vi "HFRR ADV v011 new software.vi"() -> ()   [LabVIEW 2025] (continued)
                    n2588 = call "file check.vi"("file name in"=w3137) -> ("error out"=w3140:errorcluster, "file name out"=w3135:string)  [unwired: 9 in]
                    n2589 = call "FILE PATH CREATION.vi"("error in"=w3140, "FILE NAME :"=w3135) -> ("FILE OUT"=w3138:path)  [unwired: 8 in, 1 out]
                    n2590 = Concatenate Strings(w3135, ".dgf" ("Substring")) -> (w3139:string)
                    n2591 = local read "FF 2"() -> (→"Frictional Force ( N )" →"Frictional Force ( N )":dbl)
                    n2592 = Build Path(base path=w3138, name or relative path=w3139) -> (appended path=w3134:path)
                    n2593 = local read "COF 2"() -> (w3148:dbl)
                    "cof" <- w3148
                    "Coefficient of Friction" <- w3148
                    "COF 4" <- w3148
                    "Coefficient of Friction" <- w3148
                    n2594 = local read "LVDT STROKE"() -> (w3132:dbl)
                    n2595 = local read "Add up Stroke"() -> (w3130:dbl)
                    n2596 = local read "TEMP"() -> (w3151:dbl)
                    "Temp" <- w3151
                    "Temperature ( Deg C )" <- w3151
                    n2597 = local read "Humidity ( %RH )"() -> (w3150:dbl)
                    "Humidity ( %RH )" <- w3150
                    "Humidity ( %RH )" <- w3150
                    n2598 = local read "Frequency ( Hz )"() -> (w3157:dbl)
                    n2599 = local read "Elapsed time"() -> (w3182:dbl)
                    n2600 = local read "AIR TEMP"() -> (w3155:dbl)
                    n2601 = local read "PID-out"() -> (w3160:dbl)
                    n2602 = Subtract(x=w3132, y=w3130) -> (x-y=w3131:dbl)
                    n2603 = Absolute Value(x=w3131) -> (abs(x)=w3129:dbl)
                    n2604 = local write "Temperature ( Deg C )"(w3151) -> ()
                    n2605 = Number To Fractional String(number=w3129, width (-)=i16 9 ("precision (6)"), precision (6)=i16 6) -> (F-format string=w3175:string)  [unwired: 1 in]
                    n2606 = Number To Fractional String(number=w3155, width (-)=i16 9 ("precision (6)"), precision (6)=i16 3) -> (F-format string=w3174:string)  [unwired: 1 in]
                    n2607 = Number To Fractional String(number=w3151, width (-)=i16 9 ("precision (6)"), precision (6)=i16 3) -> (F-format string=w3171:string)  [unwired: 1 in]
                    n2608 = Number To Fractional String(number=w3150, width (-)=i16 9 ("precision (6)"), precision (6)=i16 3) -> (F-format string=w3168:string)  [unwired: 1 in]
                    n2609 = Number To Fractional String(number=0.0, width (-)=i16 9 ("precision (6)"), precision (6)=i16 3) -> (F-format string=w3165:string)  [unwired: 1 in]
                    n2610 = Number To Fractional String(number=w3160, width (-)=i16 9 ("precision (6)"), precision (6)=i16 3) -> (F-format string=w3161:string)  [unwired: 1 in]
                    n2611 = Number To Fractional String(number=w3157, width (-)=i16 9 ("precision (6)"), precision (6)=i16 3) -> (F-format string=w3156:string)  [unwired: 1 in]
                    n2612 = Number To Fractional String(number=w3148, width (-)=i16 9 ("precision (6)"), precision (6)=i16 6) -> (F-format string=w3183:string)  [unwired: 1 in]
                    n2613 = Number To Fractional String(number=w3182, width (-)=i16 14 ("precision (6)"), precision (6)=i16 3) -> (F-format string=w3184:string)  [unwired: 1 in]
                    n2614 = Bundle("y"=1.02, w3129, "y"=0.98) -> (w3149:cluster{"y":dbl, dbl, "y":dbl})  [unwired: 1 in]
                    n2615 = Number To Fractional String(number="Ambient Humidity :", width (-)=i16 9 ("precision (6)"), precision (6)=i16 6) -> (F-format string=w3141:string)  [unwired: 1 in]
                    n2616 = local read "RUN"() -> (w3147:bool)
                    n2617 = case shown="True" w3147 {
                      tunnel: w3149 -> [_ w3194]
                      tunnel: w3129 -> [_ w3193]
                      tunnel: w3129 -> [_ w3191]
                      tunnel: w3129 -> [_ w3192]
                      frame False {
                      }
                      frame True {
                        "Stroke ( mm )" <- w3194
                        "Stroke ( mm )" <- w3194
                        "Stroke 4" <- w3193
                        "Stroke 3" <- w3191
                        "Stroke 2" <- w3192
                        "measured_stroke" <- w3191
                      }
                    }
                    n2618 = Concatenate Strings(w3184, w3143, w3183, w3143, w3175, w3143, w3174, w3143, w3171, w3143, w3168, w3143, w3165, w3143, w3161, w3143, w3156, w3143, w3141, "\r") -> (w3181:string)
                    n2619 = call <vilib>:"Write Characters To File.vi"("append to file? (new file:F)"=TRUE, "character string"=w3181, "file path (dialog if empty)"=w3134) -> ()  [unwired: 2 in, 1 out]
                    "refresh flag" <- TRUE ("refresh flag")
                  }
                }
                n2620 = case shown="True" w3054 {
                  tunnel: w3064 -> [_ w3090]
                  tunnel: w3069 -> [_ w3100]
                  tunnel: [0.0 w3096] -> _
                  tunnel: w3063 -> [_ w3095]
                  tunnel: [0.0 w3094] -> _
                  tunnel: w3053 -> [_ w3094]
                  tunnel: w3067 -> [w3083 _]
                  frame False {
                    n2621 = local write "acq timer"(w3083) -> ()
                    n2622 = local write "Test Duration Status"(0.0 ("Test Duration Status")) -> ()
                  }
                  frame True {
                    n2623 = local read "Set Hz"() -> (w3097:dbl)
                    n2624 = local write "Elapsed time"(w3090) -> ()
                    n2625 = local read "test time"() -> (w3089:dbl)
                    n2626 = Multiply(x=w3100, y=w3097) -> (x*y=w3099:dbl)
                    n2627 = case shown="False" w3095 {
                      tunnel: w3099 -> [w3101 _]
                      tunnel: [w3101 1.0] -> w3096
                      frame False {
                        n2628 = local write "Cycles elapsed"(w3101) -> ()
                      }
                      frame True {
                      }
                    }
                    n2629 = Greater?(x=w3090, y=w3089) -> (0:w3098:bool)
                    n2630 = Subtract(x=w3089, y=w3090) -> (x-y=w3088:dbl)
                    "time" <- w3088
                    n2631 = Multiply(x=w3088, y=60.0) -> (x*y=w3087:dbl)
                    n2632 = local write "Time Remaining"(w3087) -> ()
                    n2633 = local write "Remaining Time"(w3087) -> ()
                    n2634 = case shown="True" w3098 {
                      frame False {
                      }
                      frame True {
                        n2635 = stacked-sequence {
                          frame #0 {
                            w3106 = T17."Enabled" ("Disabled")
                            w3105 = FALSE ("TEST FILE NAM,E SAVED")
                            w3107 = "" ("FILE")
                            w3108 = TRUE ("Visible")
                            n2636 = local write "Humidity"(FALSE ("Humidity")) -> ()
                            n2637 = local write "RUN"(FALSE ("OK Button 2")) -> ()
                            n2638 = local write "Heater Button"(FALSE ("Heater Button")) -> ()
                            n2639 = local write "Auto Start Test"(FALSE ("Auto Start Test")) -> ()
                            n2640 = local write "TestCompFlg"(TRUE ("StpFlg")) -> ()
                            n2641 = local read "Humidity ( %RH )"() -> (→"Rh After":dbl)
                            n2642 = property on="STOP 2" class="Bool (strict)"("Disabled"=u8 0) -> ()  [unwired: 2 in, 2 out]
                            n2643 = local read "EVENT LOG"() -> (w3113:string)
                            n2644 = call "Event Log.vi"("Content"="Test Completed", "EVENT LOG"=w3113) -> ("EVENT LOG"=w3112:string)  [unwired: 8 in, 1 out]
                            n2645 = property on="RUN" class="Bool (strict)"("Visible"=w3108) -> ()  [unwired: 2 in, 2 out]
                            n2646 = property on="Auto Start Test" class="Bool (strict)"("Visible"=w3108) -> ()  [unwired: 2 in, 2 out]
                            n2647 = local write "Batch Ref Num :"(w3107) -> ()
                            n2648 = local write "FILE"(w3107) -> ()
                            n2649 = local write "EVENT LOG"(w3112) -> ()
                            n2650 = local write "TEST FILE NAM,E SAVED"(w3105) -> ()
                            n2651 = local write "Fuel Discription :"(w3107) -> ()
                            n2652 = local write "START TEMP"(w3105) -> ()
                            n2653 = local write "Remarks :"(w3107) -> ()
                            n2654 = local write "Main Dashboard Buttons"(T1."Imaging" ("Main Dashboard Buttons")) -> ()
                            n2655 = local write "Main Tab"(T2."Adv Scar" ("Main Tab")) -> ()
                            n2656 = property on="FRICVALZ 2" class="Bool (strict)"("DisabledEnum"=w3106) -> ()  [unwired: 2 in, 2 out]
                            n2657 = property on="FRICVALZ 3" class="Bool (strict)"("DisabledEnum"=w3106) -> ()  [unwired: 2 in, 2 out]
                            n2658 = property on="FRICVALZ 4" class="Bool (strict)"("DisabledEnum"=w3106) -> ()  [unwired: 2 in, 2 out]
                          }
                          frame #1 {
                            n2659 = Wait (ms)(milliseconds to wait=u32 1500) -> ()  [unwired: 1 out]
                          }
                          frame #2 {
                            n2660 = local write "Command"("VC;0") -> ()
                          }
                          frame #3 {
                            n2661 = Wait (ms)(milliseconds to wait=u32 1500) -> ()  [unwired: 1 out]
                          }
                          frame #4 {
                            n2662 = local write "Command"("VC;0") -> ()
                          }
                          frame #5 {
                            n2663 = Wait (ms)(milliseconds to wait=u32 1500) -> ()  [unwired: 1 out]
                          }
                          frame #6 {
                            n2664 = local write "Command"("ST;0") -> ()
                          }
                          frame #7 {
                            n2665 = local write "measured_stroke"(0.0 ("measured_stroke")) -> ()
                            n2666 = Wait (ms)(milliseconds to wait=u32 1500) -> ()  [unwired: 1 out]
                          }
                          frame #8 {
                            n2667 = local write "Command"("HE;0") -> ()
                          }
                        }
                      }
                    }
                    n2668 = Divide(x=w3090, y=w3089) -> (x/y=w3093:dbl)
                    n2669 = Multiply(x=w3093, y=100.0) -> (x*y=w3091:dbl)
                    n2670 = local write "Test Duration Status"(w3091) -> ()
                  }
                }
              }
              frame #2 {
                n2671 = case shown="True" "Heater Button" {
                  tunnel: [0.0 ("output") w3217] -> w3195
                  frame False {
                    w3198 = TRUE ("tmpchk")
                    n2672 = local read "TEMP"() -> (w3199:dbl)
                    n2673 = local write "Temp ini"(w3199) -> ()
                    n2674 = local write "Reset 4"(w3198) -> ()
                    n2675 = local write "tmpchk"(w3198) -> ()
                    n2676 = local write "reinit"(TRUE ("reinit")) -> ()
                    n2677 = local write "manual temp log"(TRUE ("manual temp log")) -> ()
                  }
                  frame True {
                    # "Logic to turn off\nthe heater when \ntemp is not rising.\nTime - 60 sec\nDelta t- 5°c"
                    n2678 = local read "Temp ini"() -> (w3206:dbl)
                    n2679 = local read "Auto Start Test"() -> (w3202:bool)
                    n2680 = Less?(x=w3206, y=53.0) -> (x < y?=w3204:bool)
                    n2681 = case shown="False" w3202 {
                      frame False {
                        n2682 = local read "Set Temp"() -> (w3226:dbl)
                        n2683 = local read "TEMP"() -> (w3225:dbl)
                        n2684 = Subtract(x=w3226, y=w3225) -> (x-y=w3224:dbl)
                        n2685 = Absolute Value(x=w3224) -> (abs(x)=w3223:dbl)
                        n2686 = Less?(x=w3223, y=0.5) -> (x < y?=w3221:bool)
                        n2687 = case shown="True" w3221 {
                          tunnel: "manual temp log" -> [_ w3227]
                          frame False {
                          }
                          frame True {
                            n2688 = case shown="True" w3227 {
                              selector: w3227 -> [_ w3228]
                              frame False {
                              }
                              frame True {
                                # "#Event log"
                                n2689 = Not(x=w3228) -> (.not. x?=w3229:bool)
                                n2690 = local write "manual temp log"(w3229) -> ()
                                n2691 = local read "EVENT LOG"() -> (w3232:string)
                                n2692 = call "Event Log.vi"("Content"="Target Temperature reached", "EVENT LOG"=w3232) -> ("EVENT LOG"=w3231:string)  [unwired: 8 in, 1 out]
                                n2693 = local write "EVENT LOG"(w3231) -> ()
                              }
                            }
                          }
                        }
                      }
                      frame True {
                        n2694 = local write "manual temp log"(TRUE ("manual temp log")) -> ()
                      }
                    }
                    n2695 = And(x="tmpchk", y=w3204) -> (x .and. y?=w3207:bool)
                    n2696 = case shown="True" w3207 {
                      frame False {
                      }
                      frame True {
                        n2697 = call "Elapsed Time8"("Time Target (s)"=300.0, "Reset"="Reset 4") -> ("Time has Elapsed"=w3234:bool)  [unwired: 10 in, 7 out]
                        n2698 = flat-sequence {
                          tunnel: w3234 -> [_]
                          frame #0 {
                            n2699 = local write "Reset 4"(FALSE ("Reset 4")) -> ()
                          }
                        }
                        n2700 = case shown="True" w3234 {
                          frame False {
                          }
                          frame True {
                            n2701 = local read "Temp ini"() -> (w3241:dbl)
                            n2702 = Add(x=w3241, y=5.0) -> (x+y=w3239:dbl)
                            n2703 = local read "TEMP"() -> (w3242:dbl)
                            n2704 = Greater?(x=w3242, y=w3239) -> (0:w3240:bool)
                            n2705 = case shown="False" w3240 {
                              frame False {
                                n2706 = local write "Heater Button"(FALSE ("Heater Button")) -> ()
                              }
                              frame True {
                                n2707 = local write "tmpchk"(FALSE ("tmpchk")) -> ()
                              }
                            }
                          }
                        }
                      }
                    }
                    n2708 = local read "Set Temp"() -> (w3215:dbl)
                    n2709 = local read "TEMP"() -> (w3209:dbl)
                    n2710 = call-poly <vilib>:"PID.vi"("reinitialize? (F)"="reinit", "dt (s)"=-1.0, "process variable"=w3209, "setpoint"=w3215) -> ("output"=w3212:dbl)  [unwired: 6 in, 1 out]
                    n2711 = Subtract(x=w3215, y=w3209) -> (x-y=w3216:dbl)
                    n2712 = Add(x=w3215, y=0.5) -> (x+y=w3213:dbl)
                    n2713 = Greater Or Equal?(x=w3209, y=w3213) -> ()  [unwired: 1 out]
                    n2714 = Select(t=0.0, s=FALSE, f=w3212) -> (s? t:f=w3211:dbl)
                    "PID output" <- w3211
                    n2715 = flat-sequence {
                      tunnel: w3211 -> [w3245]
                      tunnel: [w3245] -> w3217
                      frame #0 {
                        n2716 = local write "reinit"(FALSE ("reinit")) -> ()
                      }
                    }
                    n2717 = Bundle(w3216, "output"=w3211, "TEMP"=w3209) -> ()  [unwired: 1 in, 1 out]
                  }
                }
                "PID-out" <- w3195
              }
              frame #3 {
                n2718 = local read "TEMP"() -> (w3247:dbl)
                n2719 = Greater Or Equal?(x=w3247, y="Set Temp 2") -> (x >= y?=w3252:bool)
                n2720 = case shown="True" w3252 {
                  tunnel: [FALSE TRUE] -> w3250
                  frame False {
                  }
                  frame True {
                  }
                }
                "Status 13" <- w3250
                n2721 = And(x=w3250, y="trip1 8") -> (x .and. y?=w3249:bool)
                n2722 = case shown="True" w3249 {
                  frame False {
                    n2723 = local write "Heater Trip Temp"(TRUE ("Heater Trip Temp")) -> ()
                  }
                  frame True {
                    w3255 = FALSE ("OK Button 2")
                    n2724 = case shown="True" "Heater Trip Temp" {
                      selector: "Heater Trip Temp" -> [_ w3257]
                      frame False {
                      }
                      frame True {
                        n2725 = Not(x=w3257) -> (.not. x?=w3256:bool)
                        n2726 = local read "EVENT LOG"() -> (w3260:string)
                        n2727 = local write "Heater Trip Temp"(w3256) -> ()
                        n2728 = call "Event Log.vi"("Content"="Heater Trip", "EVENT LOG"=w3260) -> ("EVENT LOG"=w3259:string)  [unwired: 8 in, 1 out]
                        n2729 = local write "EVENT LOG"(w3259) -> ()
                      }
                    }
                    n2730 = local write "RUN"(w3255) -> ()
                    n2731 = property on="Auto Start Test" class="Bool (strict)"("Value"=w3255) -> ()  [unwired: 2 in, 2 out]
                    n2732 = local write "Heater Button"(w3255) -> ()
                  }
                }
              }
            }
            n2733 = case shown="False" w2978 {
              frame False {
                n2734 = disable-structure shown="Disabled" {
                  frame Disabled {
                    n2735 = stacked-sequence {
                      frame #0 {
                        n2736 = local write "RUN"(FALSE ("OK Button 2")) -> ()
                      }
                      frame #1 {
                      }
                    }
                  }
                  frame Enabled {
                  }
                }
              }
              frame True {
              }
            }
          }
        }
        n2737 = local read "airtempflg"() -> (w2770:bool)
        n2738 = Or(x=w2770, y=w2768) -> (x .or. y?=w2771:bool)
        n2739 = Insert Into Array(array=string[] ["Air Temperature has reached set value,", "Humidity has reached set value,", "Sample Temperaturehas reached set value,", ""], index=0, new element="") -> (w2756:string[])
        n2740 = Build Array(w2761, w2760, w2759) -> (w2757:i32[])
        n2741 = disable-structure shown="Disabled" {
          disable-tunnel: w2771 -> [w2848 _]
          disable-tunnel: w2766 -> [w2847 _]
          disable-tunnel: w2764 -> [w2846 _]
          frame Disabled {
            n2742 = Compound Arithmetic op=AND(w2848, w2847, w2846) -> ()  [unwired: 1 out]
            n2743 = case shown="True" {
              selector: _ -> [_ _]
              frame False {
              }
              frame True {
                w2849 = FALSE ("autostrtflg")
                n2744 = local write "RUN"(TRUE ("RUN")) -> ()
                n2745 = local write "autostrtflg"(w2849) -> ()
                n2746 = local write "autostart"(w2849) -> ()
                n2747 = local write "String 14"(" Running....." ("String 14")) -> ()
              }
            }
          }
          frame Enabled {
          }
        }
        n2748 = for {
          tunnel: w2757 -> [w2899] mode=indexing
          tunnel: w2756 -> [w2898]
          shift-right: [w2895] -> w2755
          shift-left: "" -> [w2897]
          n2749 = Index Array(array=w2898, index=w2899) -> (element=w2896:string)
          n2750 = Concatenate Strings(w2896, w2897) -> (w2895:string)
        }
        n2751 = local write "autostart 2"(w2755) -> ()
        n2752 = local read "Reset Graph"() -> (w2744:bool)
        n2753 = case shown="True" w2744 {
          selector: w2744 -> [_ w2798]
          frame False {
          }
          frame True {
            w2812 = 0.0 ("X Scale.Range:Maximum")
            n2754 = Not(x=w2798) -> (.not. x?=w2797:bool)
            n2755 = local write "Reset Graph"(w2797) -> ()
            n2756 = property on="Electrical Contact Resistance ( % )" class="WFChart (strict)"("XScale.Maximum"=600.0 ("X Scale.Range:Maximum"), "XScale.Minimum"=0.0 ("X Scale.Range:Minimum"), "YScale.Maximum"=100.0 ("Y Scale.Range:Maximum"), "YScale.Minimum"=0.0 ("Y Scale.Range:Minimum")) -> ()  [unwired: 2 in, 2 out]
            n2757 = property on="Frictional Force ( N )" class="WFChart (strict)"("XScale.Maximum"=600.0 ("X Scale.Range:Maximum"), "XScale.Minimum"=0.0 ("X Scale.Range:Minimum"), "YScale.Maximum"=100.0 ("Y Scale.Range:Maximum"), "YScale.Minimum"=0.0 ("Y Scale.Range:Minimum")) -> ()  [unwired: 2 in, 2 out]
            n2758 = property on="Temperature ( Deg C )" class="WFChart (strict)"("XScale.Maximum"=600.0 ("X Scale.Range:Maximum"), "XScale.Minimum"=0.0 ("X Scale.Range:Minimum"), "YScale.Maximum"=100.0 ("Y Scale.Range:Maximum"), "YScale.Minimum"=0.0 ("Y Scale.Range:Minimum")) -> ()  [unwired: 2 in, 2 out]
            n2759 = property on="Humidity ( %RH )" class="WFChart (strict)"("XScale.Maximum"=600.0 ("X Scale.Range:Maximum"), "XScale.Minimum"=0.0 ("X Scale.Range:Minimum"), "YScale.Maximum"=100.0 ("Y Scale.Range:Maximum"), "YScale.Minimum"=0.0 ("Y Scale.Range:Minimum")) -> ()  [unwired: 2 in, 2 out]
            n2760 = property on="Stroke ( mm )" class="WFChart (strict)"("XScale.Maximum"=600.0 ("X Scale.Range:Maximum"), "XScale.Minimum"=0.0 ("X Scale.Range:Minimum"), "YScale.Maximum"=100.0 ("Y Scale.Range:Maximum"), "YScale.Minimum"=0.0 ("Y Scale.Range:Minimum")) -> ()  [unwired: 2 in, 2 out]
            n2761 = property on="Coefficient of Friction" class="WFChart (strict)"("XScale.Maximum"=600.0 ("X Scale.Range:Maximum"), "XScale.Minimum"=0.0 ("X Scale.Range:Minimum"), "YScale.Maximum"=100.0 ("Y Scale.Range:Maximum"), "YScale.Minimum"=0.0 ("Y Scale.Range:Minimum")) -> ()  [unwired: 2 in, 2 out]
            n2762 = property on="Electrical Contact Resistance ( % )" class="WFChart (strict)"("XScale.Minimum"=0.0 ("X Scale.Range:Minimum"), "XScale.Maximum"=600.0 ("X Scale.Range:Maximum"), "YScale.Minimum"=0.0 ("Y Scale.Range:Minimum"), "YScale.Maximum"=100.0 ("Y Scale.Range:Maximum")) -> ()  [unwired: 2 in, 2 out]
            n2763 = property on="Temperature ( Deg C )" class="WFChart (strict)"("XScale.Minimum"=0.0 ("X Scale.Range:Minimum"), "XScale.Maximum"=600.0 ("X Scale.Range:Maximum"), "YScale.Minimum"=0.0 ("Y Scale.Range:Minimum"), "YScale.Maximum"=100.0 ("Y Scale.Range:Maximum")) -> ()  [unwired: 2 in, 2 out]
            n2764 = property on="Coefficient of Friction" class="WFChart (strict)"("XScale.Minimum"=0.0 ("X Scale.Range:Minimum"), "XScale.Maximum"=600.0 ("X Scale.Range:Maximum"), "YScale.Maximum"=1.0 ("X Scale.Range:Minimum"), "YScale.Minimum"=0.0 ("X Scale.Range:Minimum")) -> ()  [unwired: 2 in, 2 out]
            n2765 = property on="Frictional Force ( N )" class="WFChart (strict)"("XScale.Maximum"=600.0 ("X Scale.Range:Maximum"), "XScale.Minimum"=w2812, "YScale.Maximum"=10.0 ("Y Scale.Range:Maximum"), "YScale.Minimum"=w2812) -> ()  [unwired: 2 in, 2 out]
            n2766 = property on="Stroke ( mm )" class="WFChart (strict)"("XScale.Maximum"=600.0 ("X Scale.Range:Maximum"), "XScale.Minimum"=0.0 ("X Scale.Range:Minimum"), "YScale.Maximum"=100.0 ("Y Scale.Range:Maximum"), "YScale.Minimum"=0.0 ("Y Scale.Range:Minimum")) -> ()  [unwired: 2 in, 2 out]
            n2767 = property on="Humidity ( %RH )" class="WFChart (strict)"("XScale.Maximum"=600.0 ("X Scale.Range:Maximum"), "XScale.Minimum"=0.0 ("X Scale.Range:Minimum"), "YScale.Maximum"=100.0 ("Y Scale.Range:Maximum"), "YScale.Minimum"=0.0 ("Y Scale.Range:Minimum")) -> ()  [unwired: 2 in, 2 out]
          }
        }
      }
      frame "Compare Files" {
        # "Elapsed time\ncof\nstroke\nAir temp\nTemp\nHumidity"
        n2768 = case shown="True" "RSTV1 2" {
          frame False {
          }
          frame True {
            n2769 = property on="Humidity ( %RH )" class="XYGraph (strict)"("Y Scale.Display Format:Precision"=u8 0 ("Y Scale.Format & Precision:Precision")) -> ()  [unwired: 2 in, 2 out]
            n2770 = property on="Humidity ( %RH )" class="XYGraph (strict)"("X Scale.Range:Minimum"=0.0, "X Scale.Range:Maximum"=75.0, "Y Scale.Range:Minimum"=48.0, "Y Scale.Range:Maximum"=58.0) -> ()  [unwired: 2 in, 2 out]
          }
        }
        n2771 = case shown="True" "RST CP 2" {
          frame False {
          }
          frame True {
            n2772 = property on="XY Graph 13" class="XYGraph (strict)"("Y Scale.Display Format:Precision"=u8 0 ("Y Scale.Format & Precision:Precision")) -> ()  [unwired: 2 in, 2 out]
            n2773 = property on="XY Graph 13" class="XYGraph (strict)"("X Scale.Range:Minimum"=0.0, "X Scale.Range:Maximum"=75.0, "Y Scale.Range:Minimum"=0.0, "Y Scale.Range:Maximum"=100.0) -> ()  [unwired: 2 in, 2 out]
          }
        }
        n2774 = case shown="True" "RST CP" {
          frame False {
          }
          frame True {
            n2775 = property on="Sample Temperature ( °C )" class="XYGraph (strict)"("Y Scale.Display Format:Precision"=u8 2 ("Y Scale.Format & Precision:Precision")) -> ()  [unwired: 2 in, 2 out]
            n2776 = property on="Sample Temperature ( °C )" class="XYGraph (strict)"("X Scale.Range:Minimum"=0.0, "X Scale.Range:Maximum"=75.0, "Y Scale.Range:Minimum"=58.0, "Y Scale.Range:Maximum"=62.0) -> ()  [unwired: 2 in, 2 out]
          }
        }
        n2777 = case shown="True" "RSTV1 3" {
          frame False {
          }
          frame True {
            n2778 = property on="Air Temperature  ( °C )" class="XYGraph (strict)"("Y Scale.Display Format:Precision"=u8 2 ("Y Scale.Format & Precision:Precision")) -> ()  [unwired: 2 in, 2 out]
            n2779 = property on="Air Temperature  ( °C )" class="XYGraph (strict)"("X Scale.Range:Minimum"=0.0 ("Y Scale.Range:Minimum"), "X Scale.Range:Maximum"=75.0 ("Y Scale.Range:Maximum"), "Y Scale.Range:Minimum"=20.0 ("X Scale.Range:Minimum"), "Y Scale.Range:Maximum"=26.0 ("X Scale.Range:Maximum")) -> ()  [unwired: 2 in, 2 out]
          }
        }
        n2780 = case shown="True" "RSTV1 4" {
          frame False {
          }
          frame True {
            n2781 = property on="Stroke ( mm )" class="XYGraph (strict)"("Y Scale.Display Format:Precision"=u8 2 ("Y Scale.Format & Precision:Precision")) -> ()  [unwired: 2 in, 2 out]
            n2782 = property on="Stroke ( mm )" class="XYGraph (strict)"("X Scale.Range:Minimum"=0.0 ("Y Scale.Range:Maximum"), "X Scale.Range:Maximum"=75.0 ("X Scale.Range:Minimum"), "Y Scale.Range:Minimum"=0.98, "Y Scale.Range:Maximum"=1.02) -> ()  [unwired: 2 in, 2 out]
          }
        }
        n2783 = case shown="True" "rstv2" {
          frame False {
          }
          frame True {
            n2784 = property on="Coefficient Of Friction" class="XYGraph (strict)"("Y Scale.Display Format:Precision"=u8 3 ("Y Scale.Format & Precision:Precision")) -> ()  [unwired: 2 in, 2 out]
            n2785 = property on="Coefficient Of Friction" class="XYGraph (strict)"("X Scale.Range:Minimum"=0.0 ("Y Scale.Range:Maximum"), "X Scale.Range:Maximum"=75.0, "Y Scale.Range:Minimum"=0.0, "Y Scale.Range:Maximum"=1.0 ("X Scale.Range:Minimum")) -> ()  [unwired: 2 in, 2 out]
          }
        }
        n2786 = case shown="True" "RST CP 3" {
          frame False {
          }
          frame True {
            n2787 = property on="Air Temp ( °C ) vs Humidity ( % RH )" class="XYGraph (strict)"("X Scale.Range:Minimum"=18.0, "X Scale.Range:Maximum"=28.0 ("X Scale.Range:Minimum"), "Y Scale.Range:Minimum"=30.0 ("X Scale.Range:Minimum"), "Y Scale.Range:Maximum"=70.0 ("X Scale.Range:Minimum")) -> ()  [unwired: 2 in, 2 out]
          }
        }
        n2788 = case shown="True" "OPEN 1" {
          frame False {
          }
          frame True {
            (unwired) 0  # existing file
            w3536 = "Choose a datalog file to open"  # prompt
            n2789 = local write "OPEN 1"(FALSE ("OPEN 1")) -> ()
            n2790 = String To Path(string="C:\\LAB-IQ\\Data\\") -> (path=w3521:path)
            n2791 = File Dialog(6:"*.dgf" ("pattern"), 7:w3536, 11:w3521) -> (0:w3519:errorcluster, 3:w3527:path)  [unwired: 4 in, 2 out]
            n2792 = Unbundle(w3519) -> ()  [unwired: 3 out]
            n2793 = Strip Path(path=w3527) -> (name=w3526:string)  [unwired: 1 out]
            n2794 = Path To String(path=w3527) -> (string=w3522:string)
            "string1" <- w3522
            n2795 = Match Pattern(string=w3526, regular expression=".dgf") -> (before substring=→"String Control":string)  [unwired: 1 in, 3 out]
            n2796 = Match Pattern(string=w3522, regular expression=".dgf" ("substring (\"\")")) -> (before substring=w3532:string)  [unwired: 1 in, 3 out]
            n2797 = Concatenate Strings(w3532, ".duf" ("Substring")) -> (w3528:string)
            n2798 = String To Path(string=w3528) -> (path=w3533:path)
            n2799 = call <vilib>:"Read Characters From File.vi"("file path (dialog if empty)"=w3533, "start of read offset (chars.:0)"=60 ("start of read offset (chars.: 0)")) -> ("character string"=→"String Control 2":string)  [unwired: 4 in, 3 out]
          }
        }
        n2800 = case shown="True" "OPEN 2" {
          frame False {
          }
          frame True {
            (unwired) 0  # existing file
            w3554 = "Choose a datalog file to open"  # prompt
            n2801 = local write "OPEN 2"(FALSE ("OPEN 1")) -> ()
            n2802 = String To Path(string="C:\\LAB-IQ\\Data\\") -> (path=w3539:path)
            n2803 = File Dialog(6:"*.dgf" ("pattern"), 7:w3554, 11:w3539) -> (0:w3537:errorcluster, 3:w3545:path)  [unwired: 4 in, 2 out]
            n2804 = Unbundle(w3537) -> ()  [unwired: 3 out]
            n2805 = Strip Path(path=w3545) -> (name=w3543:string)  [unwired: 1 out]
            n2806 = Path To String(path=w3545) -> (string=w3540:string)
            "string1 2" <- w3540
            n2807 = Match Pattern(string=w3543, regular expression=".dgf") -> (before substring=→"String Control 3":string)  [unwired: 1 in, 3 out]
            n2808 = Match Pattern(string=w3540, regular expression=".dgf" ("substring (\"\")")) -> (before substring=w3551:string)  [unwired: 1 in, 3 out]
            n2809 = Concatenate Strings(w3551, ".duf" ("Substring")) -> (w3548:string)
            n2810 = String To Path(string=w3548) -> (path=w3546:path)
            n2811 = call <vilib>:"Read Characters From File.vi"("file path (dialog if empty)"=w3546, "start of read offset (chars.:0)"=60 ("start of read offset (chars.: 0)")) -> ("character string"=→"String Control 4":string)  [unwired: 4 in, 3 out]
          }
        }
        n2812 = case shown="True" "OPEN 3" {
          frame False {
          }
          frame True {
            (unwired) 0  # existing file
            w3572 = "Choose a datalog file to open"  # prompt
            n2813 = local write "OPEN 3"(FALSE ("OPEN 1")) -> ()
            n2814 = String To Path(string="C:\\LAB-IQ\\Data\\") -> (path=w3557:path)
            n2815 = File Dialog(6:"*.dgf" ("pattern"), 7:w3572, 11:w3557) -> (0:w3555:errorcluster, 3:w3563:path)  [unwired: 4 in, 2 out]
            n2816 = Unbundle(w3555) -> ()  [unwired: 3 out]
            n2817 = Strip Path(path=w3563) -> (name=w3561:string)  [unwired: 1 out]
            n2818 = Path To String(path=w3563) -> (string=w3558:string)
            "string1 3" <- w3558
            n2819 = Match Pattern(string=w3561, regular expression=".dgf") -> (before substring=→"String Control 5":string)  [unwired: 1 in, 3 out]
            n2820 = Match Pattern(string=w3558, regular expression=".dgf" ("substring (\"\")")) -> (before substring=w3568:string)  [unwired: 1 in, 3 out]
            n2821 = Concatenate Strings(w3568, ".duf" ("Substring")) -> (w3565:string)
            n2822 = String To Path(string=w3565) -> (path=w3569:path)
            n2823 = call <vilib>:"Read Characters From File.vi"("file path (dialog if empty)"=w3569, "start of read offset (chars.:0)"=60 ("start of read offset (chars.: 0)")) -> ("character string"=→"String Control 6":string)  [unwired: 4 in, 3 out]
          }
        }
        n2824 = case shown="True" "OPEN 4" {
          frame False {
          }
          frame True {
            (unwired) 0  # existing file
            w3590 = "Choose a datalog file to open"  # prompt
            n2825 = local write "OPEN 4"(FALSE ("OPEN 1")) -> ()
            n2826 = String To Path(string="C:\\LAB-IQ\\Data\\") -> (path=w3575:path)
            n2827 = File Dialog(6:"*.dgf" ("pattern"), 7:w3590, 11:w3575) -> (0:w3573:errorcluster, 3:w3581:path)  [unwired: 4 in, 2 out]
            n2828 = Unbundle(w3573) -> ()  [unwired: 3 out]
            n2829 = Strip Path(path=w3581) -> (name=w3579:string)  [unwired: 1 out]
            n2830 = Path To String(path=w3581) -> (string=w3576:string)
            "string1 4" <- w3576
            n2831 = Match Pattern(string=w3579, regular expression=".dgf") -> (before substring=→"String Control 7":string)  [unwired: 1 in, 3 out]
            n2832 = Match Pattern(string=w3576, regular expression=".dgf" ("substring (\"\")")) -> (before substring=w3586:string)  [unwired: 1 in, 3 out]
            n2833 = Concatenate Strings(w3586, ".duf" ("Substring")) -> (w3583:string)
            n2834 = String To Path(string=w3583) -> (path=w3587:path)
            n2835 = call <vilib>:"Read Characters From File.vi"("file path (dialog if empty)"=w3587, "start of read offset (chars.:0)"=60 ("start of read offset (chars.: 0)")) -> ("character string"=→"String Control 8":string)  [unwired: 4 in, 3 out]
          }
        }
      }
      frame "About" {
        # "Elapsed time\ncof\nstroke\nmean pos\nTemp\nHumidity"
        n2836 = disable-structure shown="Disabled" {
          frame Disabled {
            n2837 = case shown="True" "Export" {
              frame False {
              }
              frame True {
                w3612 = "                                      " ("string")
                w3614 = "\r"
                (unwired) i16 6 ("width (-)")
                w3691 = "\r"
                w3623 = "\r"
                n2838 = local write "Export"(FALSE ("Export")) -> ()
                n2839 = local read "String 29"() -> (w3660:string)
                n2840 = local read "String 34"() -> (w3648:string)
                n2841 = local read "String 35"() -> (w3643:string)
                n2842 = local read "String 37"() -> (w3639:string)
                n2843 = local read "String 36"() -> (w3636:string)
                n2844 = local read "String 38"() -> (w3633:string)
                n2845 = local read "String 39"() -> (w3630:string)
                n2846 = Match Pattern(string=w3660, regular expression=".dwm") -> (before substring=w3656:string)  [unwired: 1 in, 3 out]
                "before substring" <- w3656
                n2847 = local read "S 38"() -> (w3651:string)
                n2848 = local read "S 39"() -> (w3644:string)
                n2849 = local read "Temperature before test 2"() -> (w3680:dbl)
                n2850 = local read "Temperature after test 2"() -> (w3685:dbl)
                n2851 = local read "Humidity before test 2"() -> (w3666:dbl)
                n2852 = local read "Humidity after test 2"() -> (w3681:dbl)
                n2853 = local read "MWSD 2"() -> (w3677:dbl)
                n2854 = local read "WS1.4 2"() -> (w3693:dbl)
                n2855 = local read "HCF 2"() -> (w3689:dbl)
                n2856 = local read "AVP 2"() -> (w3678:dbl)
                n2857 = Concatenate Strings("1," ("string"), w3651) -> (w3650:string)
                n2858 = Concatenate Strings("2," ("string"), w3648) -> (w3647:string)
                n2859 = Concatenate Strings("3," ("string"), w3644) -> (w3646:string)
                n2860 = Concatenate Strings("4," ("string"), w3643) -> (w3642:string)
                n2861 = Concatenate Strings("5," ("string"), w3639) -> (w3640:string)
                n2862 = Concatenate Strings("6," ("string"), w3636) -> (w3637:string)
                n2863 = Concatenate Strings("7," ("string"), w3633) -> (w3634:string)
                n2864 = Concatenate Strings("8," ("string"), w3630) -> (w3631:string)
                n2865 = local read "Sample ID"() -> (w3698:string)
                n2866 = case shown="\"xlx\"" "Select File Type" {
                  tunnel: w3656 -> [w3701 w3703 w3705]
                  tunnel: [w3699 w3704 w3706] -> w3655
                  frame "xlx" {
                    n2867 = Concatenate Strings(w3701, ".xls" ("string")) -> (w3699:string)
                  }
                  frame "csv" {
                    n2868 = Concatenate Strings(w3703, ".csv" ("string")) -> (w3704:string)
                  }
                  frame "txt" {
                    n2869 = Concatenate Strings(w3705, ".txt" ("string")) -> (w3706:string)
                  }
                }
                n2870 = local read "Test Date"() -> (w3697:string)
                n2871 = local read "String 45"() -> (w3611:string)
                n2872 = local read "String 31"() -> (w3696:string)
                n2873 = local read "String 32"() -> (w3695:string)
                n2874 = local read "TITTLE"() -> (w3619:string)
                n2875 = Number To Fractional String(number=w3666, width (-)=i16 6, precision (6)=i16 2) -> (F-format string=w3665:string)  [unwired: 1 in]
                n2876 = Number To Fractional String(number=w3680, width (-)=i16 6, precision (6)=i16 2) -> (F-format string=w3686:string)  [unwired: 1 in]
                n2877 = Number To Fractional String(number=w3681, width (-)=i16 6, precision (6)=i16 2) -> (F-format string=w3679:string)  [unwired: 1 in]
                n2878 = Number To Fractional String(number=w3685, width (-)=i16 6, precision (6)=i16 2) -> (F-format string=w3684:string)  [unwired: 1 in]
                n2879 = Number To Fractional String(number=w3677, width (-)=i16 6, precision (6)=i16 2) -> (F-format string=w3675:string)  [unwired: 1 in]
                n2880 = Number To Fractional String(number=w3678, width (-)=i16 6, precision (6)=i16 2) -> (F-format string=w3676:string)  [unwired: 1 in]
                n2881 = Number To Fractional String(number=w3689, width (-)=i16 6, precision (6)=i16 2) -> (F-format string=w3690:string)  [unwired: 1 in]
                n2882 = Number To Fractional String(number=w3693, precision (6)=i16 2) -> (F-format string=w3694:string)  [unwired: 2 in]
                n2883 = local read "s.NO"() -> (w3613:string)
                n2884 = Concatenate Strings("=" ("string"), w3619) -> (w3618:string)
                n2885 = Concatenate Strings("S.No," ("string"), "                                       Parameters" ("string")) -> (w3624:string)
                n2886 = Concatenate Strings(w3691, w3650, w3665, w3691, w3647, w3686, w3691, w3646, w3679, w3691, w3642, w3684, w3691, w3640, w3675, w3691, w3637, w3676, w3691, w3634, w3690, w3691, w3631, w3694) -> (w3653:string)
                n2887 = Concatenate Strings(w3623, "," ("string"), w3611, w3613, w3612, w3695, w3698, w3612, w3696, w3697, w3623) -> (w3621:string)
                n2888 = local read "Tested by"() -> (w3627:string)
                n2889 = local read "String 33"() -> (w3628:string)
                n2890 = Concatenate Strings("," ("string"), "                                                                             " ("string")) -> (w3616:string)
                n2891 = Concatenate Strings(w3618, w3614, w3621, w3614, w3624, w3653, w3614, w3616, w3628, w3627) -> (→"export":string)
                n2892 = String To Path(string=w3655) -> (path=w3662:path)
                n2893 = local read "export"() -> (w3657:string)
                n2894 = call <vilib>:"Write Characters To File.vi"("append to file? (new file:F)"=FALSE, "character string"=w3657, "file path (dialog if empty)"=w3662) -> ()  [unwired: 2 in, 1 out]
              }
            }
          }
          frame Enabled {
          }
        }
        n2895 = case shown="True" "OK Button 17" {
          frame False {
          }
          frame True {
            (unwired) 0  # existing file
            w3915 = "Choose a datalog file to open"  # prompt
            n2896 = local write "OK Button 17"(FALSE ("OK Button 17")) -> ()
            n2897 = local read "String"() -> (w3910:string)
            n2898 = String To Path(string=w3910) -> (path=w3911:path)
            n2899 = File Dialog(6:"*.duf" ("pattern"), 7:w3915, 11:w3911) -> (0:w3902:errorcluster, 3:w3921:path)  [unwired: 4 in, 2 out]
            n2900 = Unbundle(w3902) -> ()  [unwired: 3 out]
            n2901 = Open/Create/Replace File "Open File"(file path (use dialog)=w3921) -> (refnum out=w3913:refnum<file>)  [unwired: 5 in, 2 out]
            n2902 = Strip Path(path=w3921) -> (name=w3919:string)  [unwired: 1 out]
            n2903 = Path To String(path=w3921) -> (string=w3904:string)
            n2904 = while {
              tunnel: w3913 -> [w3925]
              i -> [w3922]
              stop <- w3923 continue-if-true
              (unwired) TRUE ("line mode (F)")
              n2905 = Read from Text File "Read File"(file (use dialog)=w3925) -> (text=w3924:string)  [unwired: 3 in, 3 out]
              n2906 = local write "Numeric 16"(w3922) -> ()
              n2907 = String Length(string=w3924) -> (length=w3927:i32)
              n2908 = Greater?(x=w3927, y=1) -> (0:w3923:bool)
            }
            n2909 = local write "String 29"(w3904) -> ()
            n2910 = Search and Replace String(input string=w3904, search string=".duf", replace string=".dgf" ("replace string (\"\")")) -> (result string=→"String Indicator 4":string)  [unwired: 5 in, 3 out]
            n2911 = Match Pattern(string=w3919, regular expression=".dwm") -> (before substring=w3903:string)  [unwired: 1 in, 3 out]
            "String Indicator" <- w3903
            n2912 = Match Pattern(string=w3904, regular expression=".dwm" ("substring (\"\")")) -> (before substring=w3905:string)  [unwired: 1 in, 3 out]
            "String Indicator 3" <- w3905
            n2913 = local write "TITTLE 2"(w3903) -> ()
            n2914 = String To Path(string=w3905) -> (path=w3912:path)
            "path" <- w3912
            n2915 = call <vilib>:"Read Characters From File.vi"("file path (dialog if empty)"=w3912, "start of read offset (chars.:0)"=60 ("start of read offset (chars.: 0)")) -> ("character string"=→"String Indicator 2":string)  [unwired: 4 in, 3 out]
          }
        }
        n2916 = call <vilib>:"Query Available Printers.vi"() -> ("system configured printers"=w3604:string[])  [unwired: 9 in, 2 out]
        "System Configured Printers 2" <- w3604
        n2917 = local read "OK Button 16"() -> (w3601:bool)
        n2918 = case shown="True" "OK Button 16" {
          frame False {
          }
          frame True {
            n2919 = stacked-sequence {
              frame #0 {
                n2920 = local read "Numeric 16"() -> (w3929:i32)
                n2921 = local write "Numeric 10"(w3929) -> ()
              }
              frame #1 {
                n2922 = local read "S.NO"() -> (→"s.NO":string)
                n2923 = local read "String 29"() -> (w3933:string)
                n2924 = String To Path(string=w3933) -> (path=w3932:path)
                n2925 = Open/Create/Replace File "Open File"(file path (use dialog)=w3932) -> (refnum out=w3934:refnum<file>)  [unwired: 5 in, 2 out]
                n2926 = for {
                  N: 16 -> [_]
                  tunnel: w3934 -> [w3941]
                  i -> [w3937]
                  (unwired) TRUE ("line mode (F)")
                  n2927 = Read from Text File "Read File"(file (use dialog)=w3941) -> (text=w3935:string)  [unwired: 3 in, 3 out]
                  n2928 = Match Pattern(string=w3935, regular expression="(") -> (after substring=w3940:string)  [unwired: 1 in, 3 out]
                  n2929 = Match Pattern(string=w3940, regular expression=")") -> (before substring=w3936:string)  [unwired: 1 in, 3 out]
                  n2930 = case shown="1" w3937 {
                    tunnel: w3936 -> [w3942 w3943 _ _ w3944 w3945 w3946 w3948 w3950 w3952 w3954 w3956 w3958 w3960 _]
                    tunnel: w3935 -> [_ _ _ _ _ _ _ _ _ _ _ _ _ _ _]
                    frame 0 {
                      "TITTLE" <- w3942
                    }
                    frame 1 {
                      "Sample ID" <- w3943
                    }
                    frame 2 {
                    }
                    frame 3 {
                    }
                    frame 4 {
                      "Test Date" <- w3944
                    }
                    frame 5 {
                      "Tested by" <- w3945
                    }
                    frame 6 {
                      n2931 = Fract/Exp String To Number(string=w3946) -> (number=→"Humidity before test 2":dbl)  [unwired: 3 in, 1 out]
                    }
                    frame 7 {
                      n2932 = Fract/Exp String To Number(string=w3948) -> (number=→"Temperature before test 2":dbl)  [unwired: 3 in, 1 out]
                    }
                    frame 8 {
                      n2933 = Fract/Exp String To Number(string=w3950) -> (number=→"Humidity after test 2":dbl)  [unwired: 3 in, 1 out]
                    }
                    frame 9 {
                      n2934 = Fract/Exp String To Number(string=w3952) -> (number=→"Temperature after test 2":dbl)  [unwired: 3 in, 1 out]
                    }
                    frame 10 {
                      n2935 = Fract/Exp String To Number(string=w3954) -> (number=→"MWSD 2":dbl)  [unwired: 3 in, 1 out]
                    }
                    frame 11 {
                      n2936 = Fract/Exp String To Number(string=w3956) -> (number=→"AVP 2":dbl)  [unwired: 3 in, 1 out]
                    }
                    frame 12 {
                      n2937 = Fract/Exp String To Number(string=w3958) -> (number=→"HCF 2":dbl)  [unwired: 3 in, 1 out]
                    }
                    frame 13 {
                      n2938 = Fract/Exp String To Number(string=w3960) -> (number=→"WS1.4 2":dbl)  [unwired: 3 in, 1 out]
                    }
                    frame 14, Default {
                    }
                  }
                }
              }
              frame #2 {
              }
            }
            n2939 = local write "OK Button 16"(FALSE ("OK Button 13")) -> ()
          }
        }
        n2940 = Index Array(array=w3604, index="Select Printer 3") -> (element=w3606:string)
        "Selected Printer" <- w3606
        n2941 = case shown="True" w3601 {
          frame False {
          }
          frame True {
            n2942 = flat-sequence {
              frame #0 {
              }
              frame #1 {
                n2943 = Wait (ms)(milliseconds to wait=u32 100) -> ()  [unwired: 1 out]
              }
              frame #2 {
                n2944 = local write "OK Button 16"(FALSE ("Print 3")) -> ()
              }
            }
          }
        }
        n2945 = case shown="True" "Print" {
          tunnel: w3606 -> [_ w3898]
          frame False {
          }
          frame True {
            (unwired) i16 6 ("width (-)")
            (unwired) "TESTED BY : "
            (unwired) "TESTED DATE :"
            (unwired) "SAMPLE ID : "
            (unwired) "SAMPLE DESIGN : "
            w3856 = "\r"
            w3873 = "\r"
            # "add image"
            n2946 = local read "Sample ID"() -> (w3846:string)
            n2947 = local read "Tested by"() -> (w3849:string)
            n2948 = local read "String 34"() -> (w3836:string)
            n2949 = local read "String 45"() -> (w3816:string)
            n2950 = local read "String 35"() -> (w3831:string)
            n2951 = local read "String 37"() -> (w3829:string)
            n2952 = local read "String 32"() -> (w3851:string)
            n2953 = local read "String 36"() -> (w3826:string)
            n2954 = local read "String 31"() -> (w3850:string)
            n2955 = local read "Test Date"() -> (w3847:string)
            n2956 = local read "String 33"() -> (w3852:string)
            n2957 = local read "String 38"() -> (w3822:string)
            n2958 = local read "String 39"() -> (w3819:string)
            n2959 = local write "Print"(FALSE ("Print FF")) -> ()
            n2960 = local read "S 39"() -> (w3834:string)
            n2961 = local read "S 38"() -> (w3841:string)
            n2962 = local read "Temperature before test 2"() -> (w3872:dbl)
            n2963 = local read "Temperature after test 2"() -> (w3862:dbl)
            n2964 = local read "Humidity before test 2"() -> (w3887:dbl)
            n2965 = local read "Humidity after test 2"() -> (w3871:dbl)
            n2966 = local read "MWSD 2"() -> (w3876:dbl)
            n2967 = local read "WS1.4 2"() -> (w3854:dbl)
            n2968 = Concatenate Strings("2)" ("string"), w3836) -> (w3837:string)
            n2969 = Concatenate Strings("3)" ("string"), w3834) -> (w3835:string)
            n2970 = Concatenate Strings("1)" ("string"), w3841) -> (w3840:string)
            n2971 = Concatenate Strings("4)" ("string"), w3831) -> (w3832:string)
            n2972 = Concatenate Strings("5)" ("string"), w3829) -> (w3828:string)
            n2973 = Concatenate Strings("6)" ("string"), w3826) -> (w3825:string)
            n2974 = Concatenate Strings("7)" ("string"), w3822) -> (w3823:string)
            n2975 = Concatenate Strings("8)" ("string"), w3819) -> (w3820:string)
            n2976 = local read "HCF 2"() -> (w3858:dbl)
            n2977 = local read "AVP 2"() -> (w3875:dbl)
            n2978 = local read "s.NO"() -> (w3817:string)
            n2979 = call <vilib>:"New Report.vi"("report type"=enum16{"Standard Report", "HTML"}."Standard Report") -> ("report out"=w3896:refnum<class "NI_report.lvclass">, "error out"=w3895:errorcluster)  [unwired: 13 in]
            n2980 = local read "TITTLE"() -> (w3848:string)
            n2981 = Concatenate Strings(w3873, w3816, w3817, w3873, w3851, w3846, w3873, w3850, w3847, w3873, w3852, w3849, w3873) -> (w3866:string)
            "test by" <- w3866
            n2982 = Number To Fractional String(number=w3872, width (-)=i16 6, precision (6)=i16 2) -> (F-format string=w3861:string)  [unwired: 1 in]
            n2983 = Number To Fractional String(number=w3871, width (-)=i16 6, precision (6)=i16 2) -> (F-format string=w3874:string)  [unwired: 1 in]
            n2984 = Number To Fractional String(number=w3887, width (-)=i16 6, precision (6)=i16 2) -> (F-format string=w3892:string)  [unwired: 1 in]
            n2985 = Number To Fractional String(number=w3876, width (-)=i16 6, precision (6)=i16 2) -> (F-format string=w3878:string)  [unwired: 1 in]
            n2986 = Number To Fractional String(number=w3862, width (-)=i16 6, precision (6)=i16 2) -> (F-format string=w3863:string)  [unwired: 1 in]
            n2987 = Number To Fractional String(number=w3875, width (-)=i16 6, precision (6)=i16 2) -> (F-format string=w3877:string)  [unwired: 1 in]
            n2988 = Number To Fractional String(number=w3858, width (-)=i16 6, precision (6)=i16 2) -> (F-format string=w3857:string)  [unwired: 1 in]
            n2989 = Number To Fractional String(number=w3854, precision (6)=i16 2) -> (F-format string=w3853:string)  [unwired: 2 in]
            n2990 = call-dynamic "Set Report Header Text.vi"("report in"=w3896, "center header text"=w3848, "error in (no error)"=w3895) -> ("report out"=w3867:refnum<class "NI_report.lvclass">, "error out"=w3868:errorcluster)  [unwired: 11 in]
            n2991 = Concatenate Strings(w3856, w3840, w3892, w3856, w3837, w3861, w3856, w3835, w3874, w3856, w3832, w3863, w3856, w3828, w3878, w3856, w3825, w3877, w3856, w3823, w3857, w3856, w3820, w3853) -> (w3844:string)
            "export 2" <- w3844
            n2992 = call-poly <vilib>:"Append Report Text.vi"("report in"=w3867, "text"=w3866, "error in (no error)"=w3868) -> ("report out"=w3870:refnum<class "NI_report.lvclass">, "error out"=w3869:errorcluster)  [unwired: 9 in, 2 out]
            n2993 = local read "test by"() -> (w3843:string)
            n2994 = local read "TITTLE"() -> (w3845:string)
            n2995 = call-poly <vilib>:"Append Report Text.vi"("report in"=w3870, "error in (no error)"=w3869) -> ("report out"=w3891:refnum<class "NI_report.lvclass">, "error out"=w3889:errorcluster)  [unwired: 10 in, 2 out]
            n2996 = Concatenate Strings(w3845, w3844, w3843) -> (→"output":string)
            n2997 = call-poly <vilib>:"Append Report Text.vi"("report in"=w3891, "text"=w3844, "error in (no error)"=w3889) -> ("report out"=w3890:refnum<class "NI_report.lvclass">, "error out"=w3888:errorcluster)  [unwired: 9 in, 2 out]
            n2998 = call-dynamic "Print Report.vi"("report in"=w3890, "printer name (default)"=w3898, "error in (no error)"=w3888) -> ("report out"=w3900:refnum<class "NI_report.lvclass">, "error out"=w3901:errorcluster)  [unwired: 11 in]
            n2999 = call-dynamic "Dispose Report.vi"("report in"=w3900, "error in (no error)"=w3901) -> ()  [unwired: 13 in, 1 out]
          }
        }
        n3000 = case shown="True" "Print 2" {
          frame False {
          }
          frame True {
            n3001 = flat-sequence {
              frame #0 {
                n3002 = local read "s.NO"() -> (→"s.NO 2":string)
                n3003 = Wait (ms)(milliseconds to wait=u32 20) -> ()  [unwired: 1 out]
                n3004 = local read "Sample ID  3"() -> (→"Sample ID  6":string)
                n3005 = local read "Sample ID  4"() -> (→"Sample ID  7":string)
                n3006 = local read "Sample ID"() -> (→"Sample ID  2":string)
                n3007 = local read "Tested by"() -> (→"Tested by 2":string)
                n3008 = local read "Test Date"() -> (→"Test Date 2":string)
                n3009 = local read "Humidity after test 3"() -> (→"Humidity after test 4":dbl)
                n3010 = local read "Ref A Test Date :"() -> (→"TITTLE 4":string)
                n3011 = local read "Temperature before test 3"() -> (w3723:dbl)
                n3012 = local read "Temperature before test 3"() -> (→"Temperature after test 5":dbl)
                n3013 = local read "Temperature after test 3"() -> (→"Temperature after test 4":dbl)
                n3014 = local read "Humidity before test 3"() -> (→"Humidity before test 4":dbl)
                n3015 = local write "Temperature before test 3"(w3723) -> ()
                n3016 = local read "image data"() -> (w3714:T15)
                n3017 = String To Path(string="C:\\LAB-IQ\\im\\Temp_resized.jpg") -> (path=w3715:path)
                "path 2" <- w3715
                n3018 = call <vilib>:"Write JPEG File.vi"("image data"=w3714, "path to JPEG file"=w3715) -> ()  [unwired: 8 in, 2 out]
                "Ref A Test Date :" <- "Ref A Test Date :"
                "Ref B Test Date :" <- "Ref B Test Date :"
                "Ref B Scar Value :" <- "Ref B Scar Value :"
                "Ref A Scar Value :" <- "Ref A Scar Value :"
              }
              frame #1 {
                (unwired) HTML_Report_Image_Alignment."MIDDLE" ("alignment (default)")
                w3751 = u16 0 items=["portrait", "landscape"] ("orientation (portrait)")
                (unwired) HTML_Report_Image_Alignment."ABSMIDDLE" ("alignment (default)")
                (unwired) "TESTED BY : "
                (unwired) "TESTED DATE :"
                (unwired) "SAMPLE ID : "
                (unwired) "SAMPLE DESIGN : "
                w3784 = "\r"
                # "add image"
                n3019 = Wait (ms)(milliseconds to wait=u32 20) -> ()  [unwired: 1 out]
                n3020 = local read "Sample ID  2"() -> (w3777:string)
                n3021 = local read "Wear Scar X"() -> (w3749:dbl)
                "Length ( microns ) 2" <- w3749
                n3022 = local read "Wear Scar Y"() -> (w3748:dbl)
                "Wear Scar Y ( microns ) :" <- w3748
                n3023 = local read "Test Date 2"() -> (w3778:string)
                n3024 = local read "Tested by 2"() -> (w3779:string)
                n3025 = local read "String 46"() -> (w3775:string)
                n3026 = local read "String 48"() -> (w3781:string)
                n3027 = local read "String 47"() -> (w3780:string)
                n3028 = local read "String 49"() -> (w3782:string)
                n3029 = local read "String 10"() -> (w3735:string)
                n3030 = local read "s.NO 2"() -> (w3776:string)
                n3031 = Add(x=w3749, y=w3748) -> (x+y=w3747:dbl)
                n3032 = call <vilib>:"New Report.vi"("report type"=enum16{"Standard Report", "HTML"}."HTML") -> ("report out"=w3755:refnum<class "NI_report.lvclass">, "error out"=w3753:errorcluster)  [unwired: 13 in]
                n3033 = Concatenate Strings(w3784, w3775, w3776, w3784, w3781, w3777, w3784, w3780, w3778, w3784, w3782, w3779, w3784) -> (→"test by 2":string)
                n3034 = Concatenate Strings("C:\\LAB-IQ\\Data\\" ("string"), w3735, ".jpg" ("string")) -> ()  [unwired: 1 out]
                n3035 = Divide(x=w3747, y=2.0) -> (x/y=→"Mean Wear ( microns) :":dbl)
                n3036 = call-dynamic "Set Report Orientation.vi"("report in"=w3755, "orientation (portrait)"=w3751, "error in (no error)"=w3753) -> ("report out"=w3754:refnum<class "NI_report.lvclass">, "error out"=w3752:errorcluster)  [unwired: 11 in]
                n3037 = for {
                  N: 5 -> [_]
                  tunnel: w3754 -> [w3805]
                  tunnel: [w3804] -> w3733
                  tunnel: w3752 -> [w3803]
                  tunnel: [w3802] -> w3732
                  n3038 = call-dynamic "Set Report Tab Width.vi"("report in"=w3805, "error in (no error)"=w3803) -> ("report out"=w3804:refnum<class "NI_report.lvclass">, "error out"=w3802:errorcluster)  [unwired: 12 in]
                }
                n3039 = local read "TITTLE"() -> (w3750:string)
                n3040 = call-dynamic "Set Report Header Text.vi"("report in"=w3733, "center header text"=w3750, "error in (no error)"=w3732) -> ("report out"=w3771:refnum<class "NI_report.lvclass">, "error out"=w3770:errorcluster)  [unwired: 11 in]
                n3041 = for {
                  N: 1 -> [_]
                  tunnel: [w3809] -> w3757
                  tunnel: [w3808] -> w3756
                  tunnel: w3771 -> [w3807]
                  tunnel: w3770 -> [w3806]
                  n3042 = call-dynamic "New Report Line.vi"("report in"=w3807, "error in (no error)"=w3806) -> ("report out"=w3809:refnum<class "NI_report.lvclass">, "error out"=w3808:errorcluster)  [unwired: 12 in]
                }
                n3043 = for {
                  N: 2 -> [_]
                  tunnel: [w3801] -> w3763
                  tunnel: [w3800] -> w3762
                  tunnel: w3757 -> [w3799]
                  tunnel: w3756 -> [w3798]
                  n3044 = call-dynamic "New Report Line.vi"("report in"=w3799, "error in (no error)"=w3798) -> ("report out"=w3801:refnum<class "NI_report.lvclass">, "error out"=w3800:errorcluster)  [unwired: 12 in]
                }
                n3045 = for {
                  N: 25 -> [_]
                  tunnel: w3763 -> [w3797]
                  tunnel: w3762 -> [w3795]
                  tunnel: [w3796] -> w3766
                  tunnel: [w3794] -> w3765
                  n3046 = call-dynamic "Set Report Tab Width.vi"("report in"=w3797, "error in (no error)"=w3795) -> ("report out"=w3796:refnum<class "NI_report.lvclass">, "error out"=w3794:errorcluster)  [unwired: 12 in]
                }
                n3047 = control-ref of="Tab Control 9"() -> (w3761:refnum<vi>)
                n3048 = call-dynamic "Append Control Image to Report.vi"("report in"=w3766, "alignment (default)"=HTML_Report_Image_Alignment."ABSMIDDLE", "ctrl reference"=w3761, "error in (no error)"=w3765) -> ("report out"=w3760:refnum<class "NI_report.lvclass">, "error out"=w3759:errorcluster)  [unwired: 8 in, 2 out]
                n3049 = for {
                  N: 3 -> [_]
                  tunnel: [w3793] -> w3744
                  tunnel: [w3792] -> w3743
                  tunnel: w3760 -> [w3791]
                  tunnel: w3759 -> [w3790]
                  n3050 = call-dynamic "New Report Line.vi"("report in"=w3791, "error in (no error)"=w3790) -> ("report out"=w3793:refnum<class "NI_report.lvclass">, "error out"=w3792:errorcluster)  [unwired: 12 in]
                }
                n3051 = for {
                  N: 100 -> [_]
                  tunnel: w3744 -> [w3789]
                  tunnel: w3743 -> [w3787]
                  tunnel: [w3788] -> w3740
                  tunnel: [w3786] -> w3738
                  n3052 = call-dynamic "Set Report Tab Width.vi"("report in"=w3789, "error in (no error)"=w3787) -> ("report out"=w3788:refnum<class "NI_report.lvclass">, "error out"=w3786:errorcluster)  [unwired: 12 in]
                }
                n3053 = String To Path(string="C:\\LAB-IQ\\im\\Temp_resized.jpg") -> (path=w3730:path)
                n3054 = call-poly <vilib>:"Append Image to Report.vi"("report in"=w3740, "path or URL of image"=w3730, "error in (no error)"=w3738) -> ("report out"=w3739:refnum<class "NI_report.lvclass">, "error out"=w3737:errorcluster)  [unwired: 9 in, 2 out]
                n3055 = call-poly <vilib>:"Open HTML Report in Browser.vi"("report in"=w3739, "error in (no error)"=w3737) -> ("report out"=w3774:refnum<class "NI_report.lvclass">, "error out"=w3773:errorcluster)  [unwired: 11 in, 1 out]
                n3056 = call-dynamic "Dispose Report.vi"("report in"=w3774, "error in (no error)"=w3773) -> ()  [unwired: 13 in, 1 out]
              }
              frame #2 {
              }
